vi "Check Blower Running.vi"(7 "Blower":T1, 8 "error in (no error)":errorcluster, 11 "cRIO-CO2 in":refnum<class "cRIO-CO2.lvclass">) -> (0 "error out":errorcluster, 1 "Running?":bool, 3 "cRIO-CO2 out":refnum<class "cRIO-CO2.lvclass">)   [LabVIEW 2015, in "cRIO-Carbondioxide.lvlib" / "cRIO-CO2.lvlib" / "cRIO-CO2.lvclass"]
uses:
  cRIO-CO2.lvclass
  Blowers Heaters Enumerator.ctl
  <vilib>/ActorFramework/Message Enqueuer/Message Priority.ctl
  cRIO-CO2.lvclass/cRIO-CO2.ctl
  CO2 Actor Messages/Ping Msg/Ping Msg.lvclass/Ping Msg.ctl
  <vilib>/ActorFramework/Message Enqueuer/Message Enqueuer.lvclass/Message Enqueuer.ctl
  <vilib>/ActorFramework/Message Enqueuer/Enqueue.vi
  <vilib>/ActorFramework/Message Priority Queue/Priority Enqueue.vi
  <vilib>/ActorFramework/Message Enqueuer/Message Enqueuer.lvclass
  CO2 Actor Messages/Ping Msg/Ping Msg.lvclass
  <vilib>/ActorFramework/Actor/Actor.lvclass
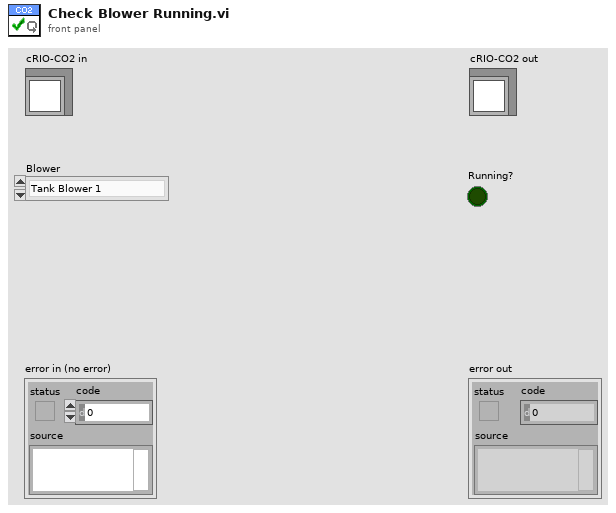
[diagram p1: front panel]
types:
  T1 = typedef "cRIO-Carbondioxide.lvlib/cRIO-CO2.lvlib/cRIO-CO2.lvclass/Blowers Heaters Enumerator.ctl" = enum16{"Tank Blower 1", "Tank Blower 2", "Tank Blower 3", "Tank Blower 4", "Syringe Blower", "Syringe Heater", "Piston Heater", "Undefined"}
  T2 = typedef "Actor Framework.lvlib/Message Enqueuer.lvclass/Message Priority.ctl" = enum16{"Low", "Normal", "High"}
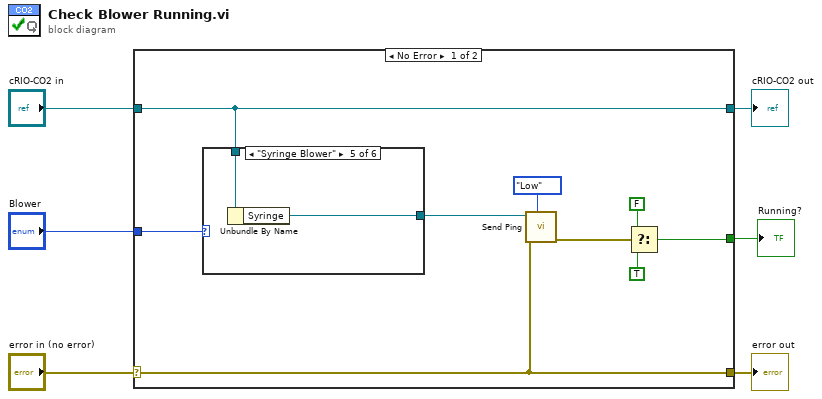
[diagram p0: block diagram]
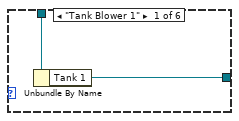
[diagram p2: hidden frame]
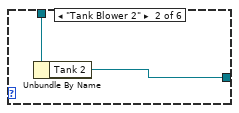
[diagram p3: hidden frame]
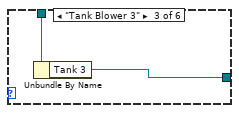
[diagram p4: hidden frame]
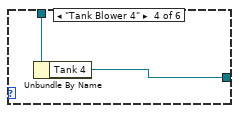
[diagram p5: hidden frame]
diagram:
  n1 = case shown="No Error" "error in (no error)" {
    selector: "error in (no error)" -> [w13 w27]
    tunnel: [w13 w27] -> w5
    tunnel: [w14 w26] -> w3
    tunnel: "cRIO-CO2 in" -> [w14 w26]
    tunnel: "Blower" -> [w15 _]
    tunnel: [w8 _] -> w1
    frame No Error {
      n2 = case shown="\"Syringe Blower\"" w15 {
        tunnel: w14 -> [w17 w19 w21 w23 w25 _]
        tunnel: [w16 w18 w20 w22 w24 _] -> w7
        frame "Tank Blower 1" {
          n3 = Unbundle By Name(w17) -> ("Tank 1"=w16:refnum<class "Message Enqueuer.lvclass">)
        }
        frame "Tank Blower 2" {
          n4 = Unbundle By Name(w19) -> ("Tank 2"=w18:refnum<class "Message Enqueuer.lvclass">)
        }
        frame "Tank Blower 3" {
          n5 = Unbundle By Name(w21) -> ("Tank 3"=w20:refnum<class "Message Enqueuer.lvclass">)
        }
        frame "Tank Blower 4" {
          n6 = Unbundle By Name(w23) -> ("Tank 4"=w22:refnum<class "Message Enqueuer.lvclass">)
        }
        frame "Syringe Blower" {
          n7 = Unbundle By Name(w25) -> ("Syringe"=w24:refnum<class "Message Enqueuer.lvclass">)
        }
        frame "Undefined", Default {
        }
      }
      n8 = call "Send Ping.vi"("Message Priority (Normal)"=Message_Priority."Low", "error in (no error)"=w13, "Message Enqueuer"=w7) -> ("error out"=w11:errorcluster)  [unwired: 5 in, 3 out]
      n9 = Select(t=FALSE, s=w11, f=TRUE) -> (s? t:f=w8:bool)
    }
    frame Error {
    }
  }
  "error out" <- w5
  "cRIO-CO2 out" <- w3
  "Running?" <- w1
